vi "Insert Type Name.vi"(7 "Pretty Print?":bool, 10 "Type Name":string, 11 "<JSON> in":string) -> (3 "<JSON> out":string)   [LabVIEW 2017, in "Flatten To JSON Object.lvclass"]
doc: "Inserts the type name at the beginning of a JSON object."
uses:
  Flatten To JSON Object.lvclass
  <vilib>/JDP Science/JSONtext/Get all Object Items.vi
  <vilib>/JDP Science/JSONtext/Set Multiple Object Items.vi
  <vilib>/JDP Science/JSONtext/JSONtext.lvlib
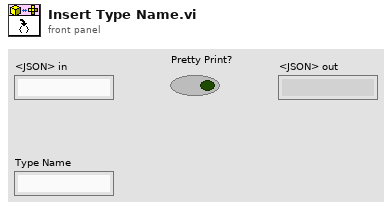
[diagram p1: front panel]
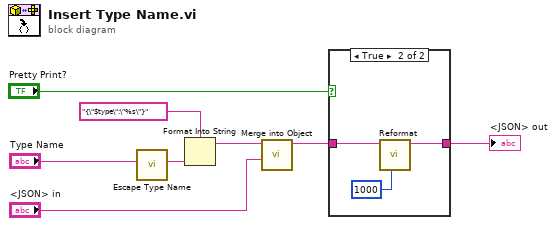
[diagram p0: block diagram]
diagram:
  n1 = call "Escape Type Name.vi"("String"="Type Name") -> ("String out"=w7:string)  [unwired: 10 in]
  n2 = Format Into String(format string="{\"$type\":\"%s\"}", w7) -> (resulting string=w1:string)  [unwired: 2 in, 1 out]
  n3 = call <vilib>:"Merge into Object.vi"("JSON Object to Merge"="<JSON> in", "JSON"=w1) -> ("<JSON>"=w3:string)  [unwired: 7 in, 1 out]
  n4 = case shown="True" "Pretty Print?" {
    tunnel: w3 -> [w9 w12]
    tunnel: [w9 w10] -> w5
    frame False {
    }
    frame True {
      n5 = call <vilib>:"Reformat.vi"("Pretty Print Levels"=1000, "JSON"=w12) -> ("<JSON>"=w10:string)  [unwired: 6 in, 3 out]
    }
  }
  "<JSON> out" <- w5
